vi "_LockState JKISMQ.vi"(8 "Error in":errorcluster caption="Error in (no error)", 11 "JKISMQ":T1) -> (0 "Error out":errorcluster, 2 "lock":bool, 3 "JKISMQ":T1)   [LabVIEW 2014, in "JKI-State-Machine-Plus.lvlib"]
uses:
  JKI-State-Machine-Plus.lvlib
  _JKISMQ.ctl
  _Cross JKI StateMachine State Data.ctl
  _Cross JKI StateMachine State Response.ctl
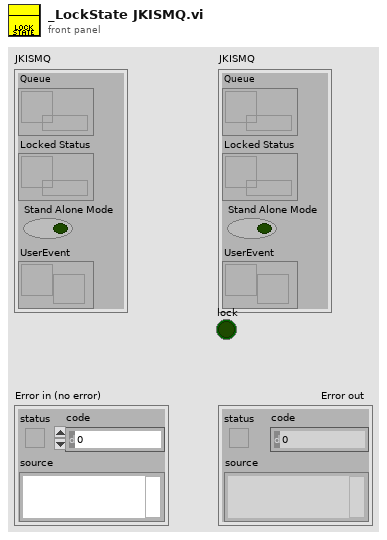
[diagram p1: front panel]
types:
  T1 = typedef "JKI-State-Machine-Plus.lvlib/_JKISMQ.ctl" = cluster{"Queue":refnum<queue>, "Locked Status":refnum<data-value>, "Stand Alone Mode":bool, "UserEvent":refnum<user-event>}
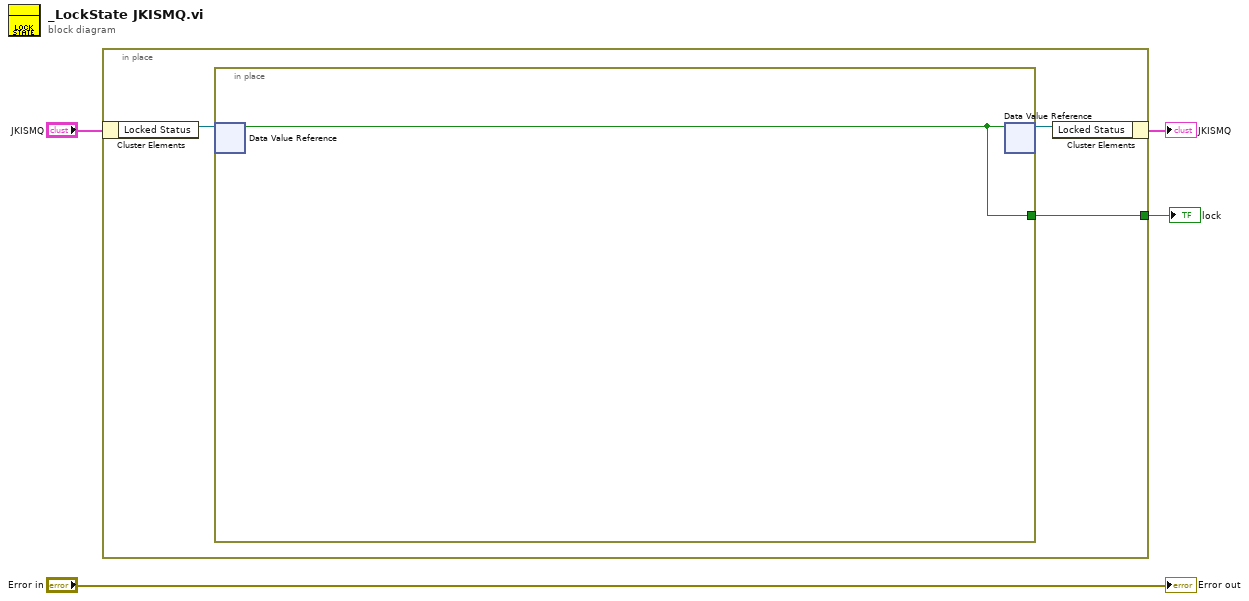
[diagram p0: block diagram]
diagram:
  n1 = in-place "In Place Element Structure" {
    in-place-border: [w5] -> w1
    n2 = in-place-cluster #1("JKISMQ") -> ("Locked Status"=w7:refnum<data-value>)
    n3 = in-place {
      in-place-border: [w8] -> w5
      n4 = in-place-dvr #2(w7) -> (w8:bool)  [unwired: 1 out]
      n5 = in-place-dvr #2(w8) -> (w6:refnum<data-value>)  [unwired: 1 out]
    }
    n6 = in-place-cluster #1("Locked Status"=w6) -> (→"JKISMQ":T1)
  }
  "lock" <- w1
  "Error out" <- "Error in"
